vi "Sting Contains.vi"(1 "Expression to evaluate":string="STOP", 2 "Input String":string) -> (0 "Boolean":bool)   [LabVIEW 2012]
doc: "This VI finds out if a string contains an expression and returns a true or false boolean."
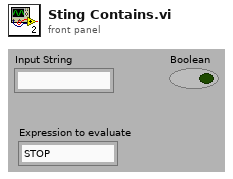
[diagram p1: front panel]
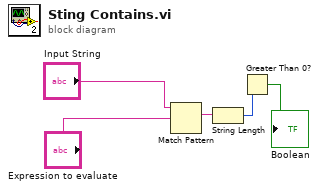
[diagram p0: block diagram]
diagram:
  n1 = Match Pattern(string="Input String", regular expression="Expression to evaluate") -> (match substring=w2:string)  [unwired: 1 in, 3 out]
  n2 = String Length(string=w2) -> (length=w4:i32)
  n3 = Greater Than 0?(x=w4) -> (x > 0?=→"Boolean":bool)
